vi "Factory Create.vi"(8 "Error In":errorcluster, 11 "reference in":refnum<class "Fetch Waveforms CFG.lvclass">) -> (0 "Error Out":errorcluster, 3 "reference out":refnum<class "Fetch Waveforms CFG.lvclass">)   [LabVIEW 2023, in "Scope Simulated.lvlib" / "Fetch Waveforms CFG.lvclass"]
uses:
  Fetch Waveforms CFG.lvclass
  Fetch Waveforms CFG.lvclass/Fetch Waveforms CFG.ctl
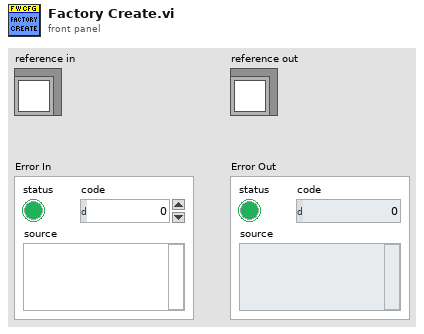
[diagram p1: front panel]
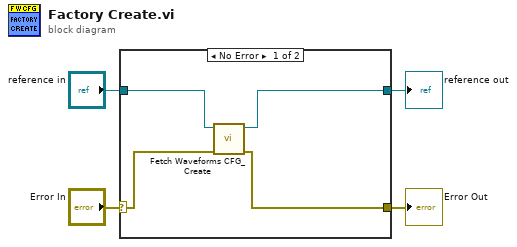
[diagram p0: block diagram]
diagram:
  n1 = case shown="No Error" "Error In" {
    selector: "Error In" -> [w6 w10]
    tunnel: [w5 w10] -> w3
    tunnel: [w7 w9] -> w1
    tunnel: "reference in" -> [w8 w9]
    frame No Error {
      n2 = call "Fetch Waveforms CFG_Create.vi"("Error In"=w6, "reference in"=w8) -> ("Error Out"=w5:errorcluster, "reference out"=w7:refnum<class "Fetch Waveforms CFG.lvclass">)  [unwired: 8 in]
    }
    frame Error {
    }
  }
  "Error Out" <- w3
  "reference out" <- w1
